vi "UTF-8 Mode Windows.vi"(8 "error in (no error)":errorcluster, 11 "ASE Handle":refnum<class "ase.lvclass">) -> (0 "error out":errorcluster, 2 "Use UTF-8 on Windows":bool)   [LabVIEW 2020, in "serenial.io-ase.lvlib" / "ase.lvclass"]
doc: "Specify the Identifier that will be used for every event from this Asynchronous System Exec Instance."
uses:
  ase.lvclass
  ase.lvclass/ase.ctl
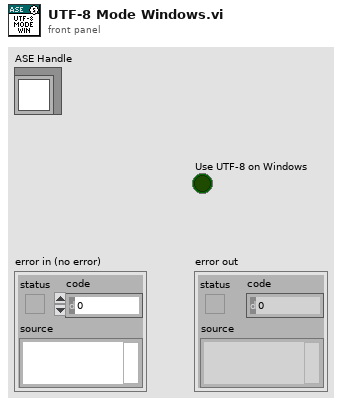
[diagram p1: front panel]
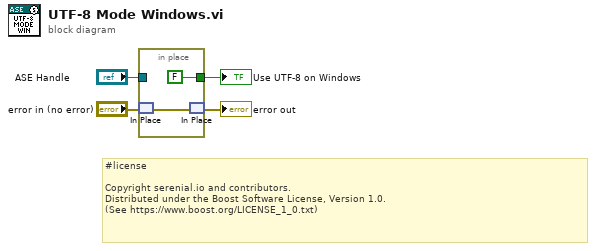
[diagram p0: block diagram]
diagram:
  # "#license\n\nCopyright serenial.io and contributors.\nDistributed under the Boost Software License, Version 1.0.\n(See https://www.boost.org/LICENSE_1_0.txt)"
  n1 = in-place "In Place Element Structure" {
    in-place-border: "ASE Handle" -> [_]
    in-place-border: [FALSE] -> w1
    n2 = in-place-match #1 ("In Place In / Out Element")("error in (no error)") -> (w6:errorcluster)
    n3 = in-place-match #1 ("In Place In / Out Element")(w6) -> (→"error out":errorcluster)
  }
  "Use UTF-8 on Windows" <- w1
